vi "Tutorial_6_Event Structure.vi"() -> ()   [LabVIEW 2020]
panel:
  out "Numeric 2":i32
  out "Numeric":i32
  out "LED 2":bool
  out "LED1":bool
  in  "S 2":bool
  in  "S1":bool
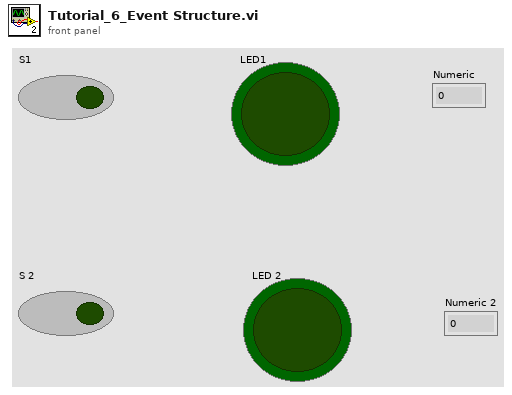
[diagram p1: front panel]
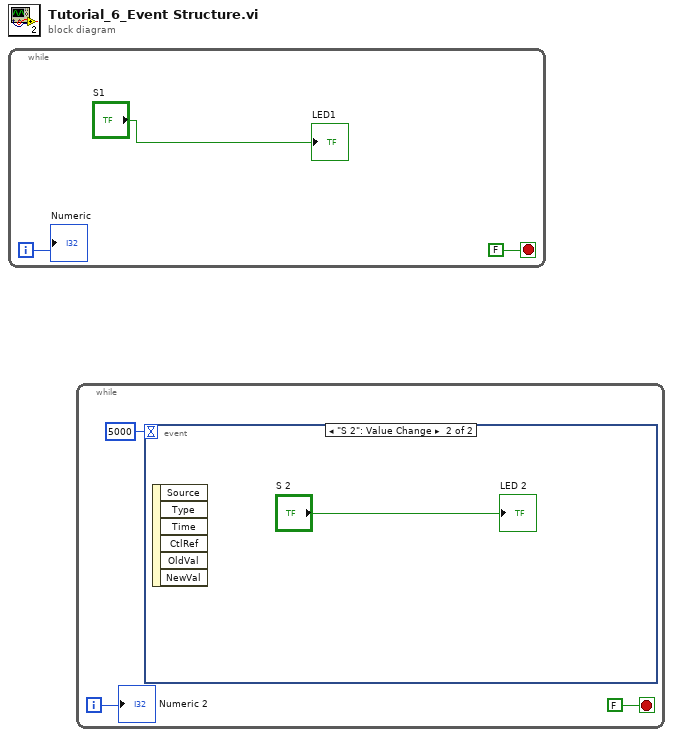
[diagram p0: block diagram]
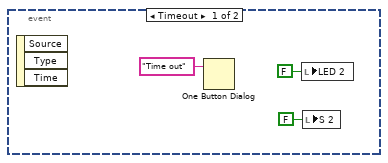
[diagram p2: hidden frame]
diagram:
  n1 = while {
    i -> [w1]
    stop <- FALSE stop-if-true
    "LED1" <- "S1"
    "Numeric" <- w1
  }
  n2 = while {
    i -> [w5]
    stop <- FALSE stop-if-true
    n3 = event shown="[1] \"S 2\": Value Change" {
      selector: _ -> [_ _]
      dyn-events: _ -> [_ _]
      timeout: 5000 -> [_ _]
      event Timeout {
        n4 = event-data() -> ()  [unwired: 1 in, 3 out]
        n5 = One Button Dialog(message="Time out") -> ()  [unwired: 1 in, 1 out]
        n6 = local write "LED 2"(FALSE ("LED 2")) -> ()
        n7 = local write "S 2"(FALSE ("S 2")) -> ()
      }
      event "S 2": Value Change {
        n8 = event-data() -> ()  [unwired: 1 in, 6 out]
        "LED 2" <- "S 2"
      }
    }
    "Numeric 2" <- w5
  }
